vi "ABB Report Bearing run.vi"(10 "Report in":string) -> (2 "Report out":string)   [LabVIEW 2017]
uses:
  ABB global.vi
panel:
  out "Selected Entries":string[](array[string])
  out "appended array":string[][](array[string])
  out "subarray":dbl[](array[numeric])
  out "Bearing run":cluster{"Heat run results":dbl[], dbl[]}[](graph)
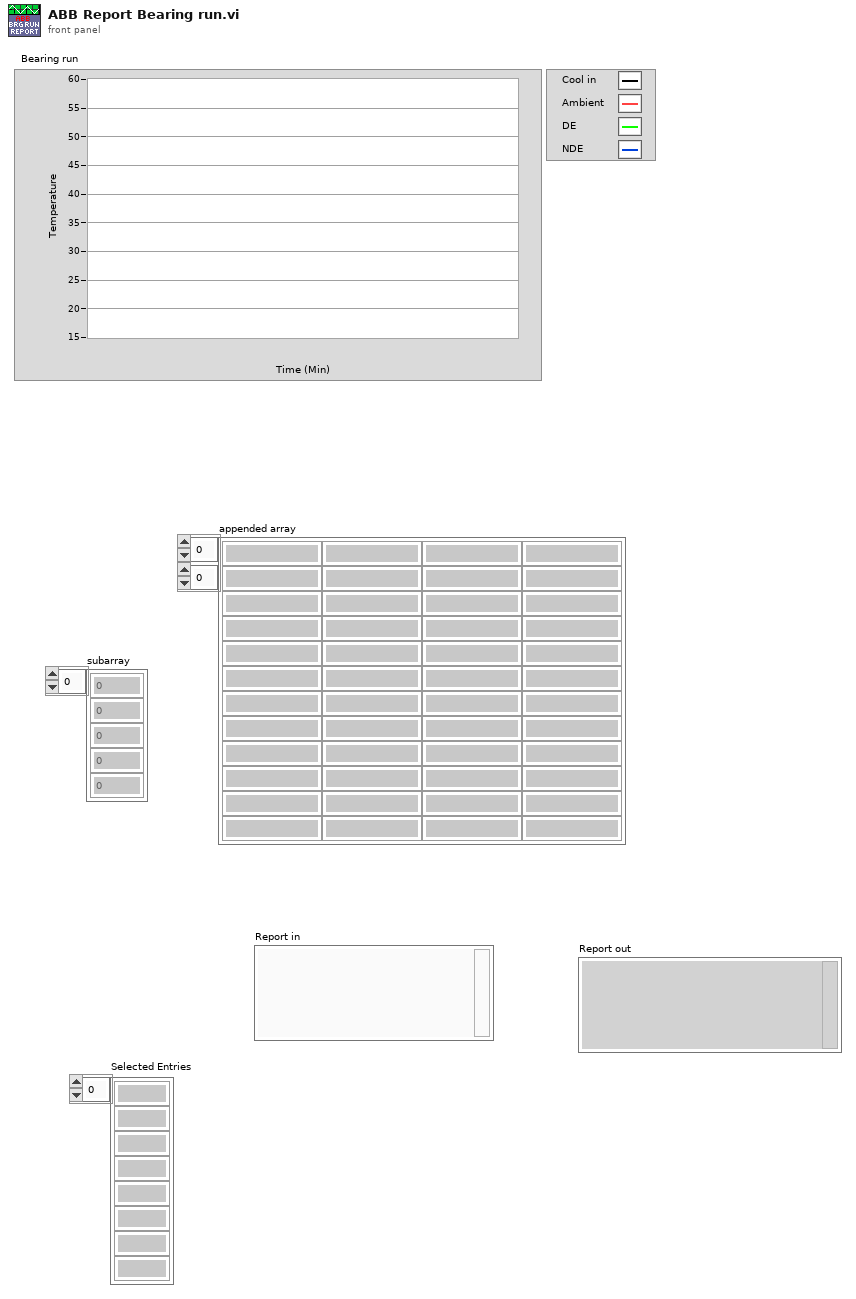
[diagram p1: front panel]
types:
  T1 = cluster{"temp. alloc":i32[], "category":i32[], "Category names":string[], "Category none names":string[]}
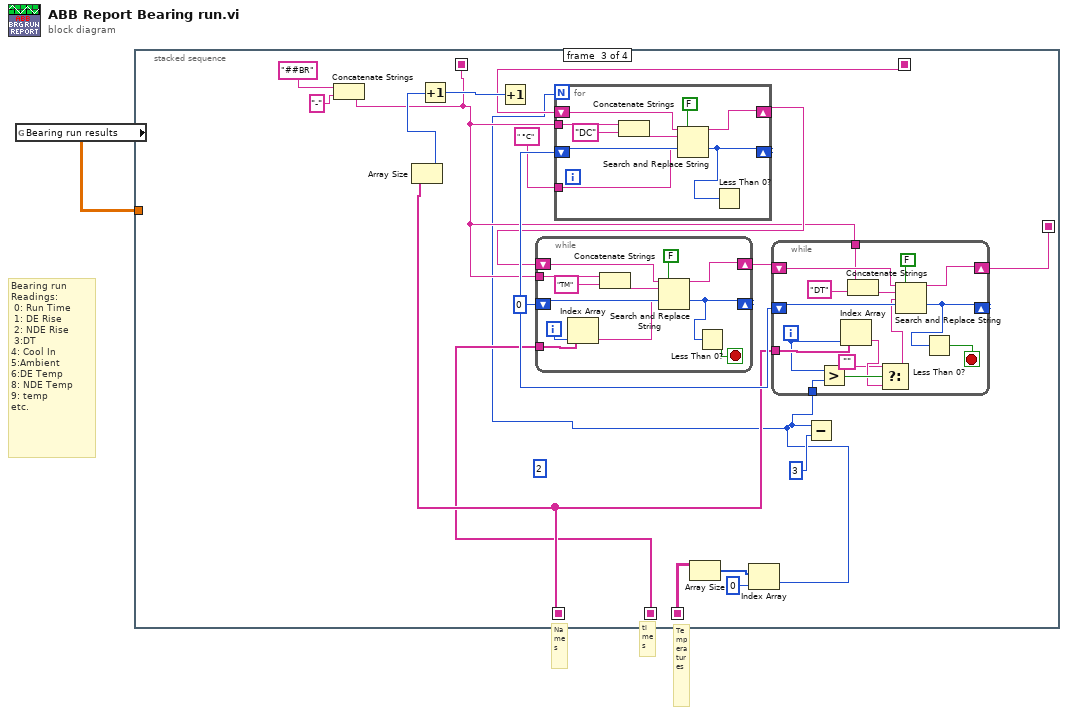
[diagram p0: block diagram]
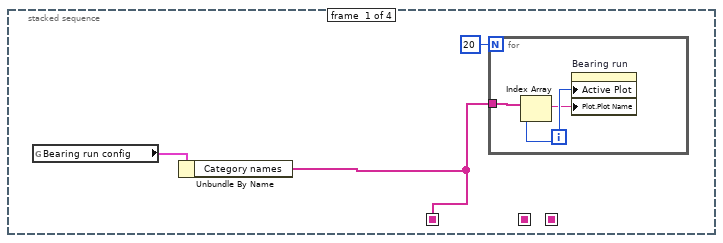
[diagram p2: hidden frame]
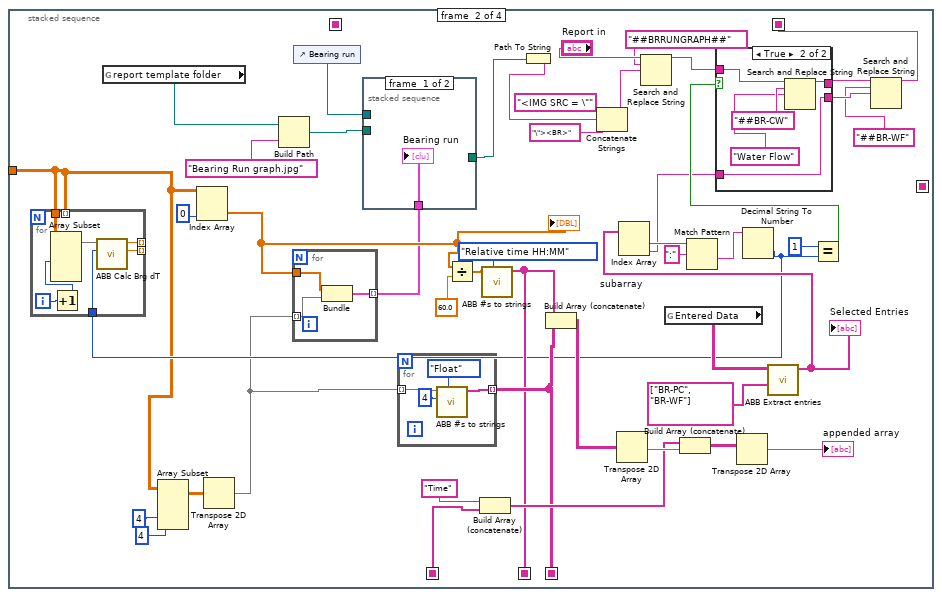
[diagram p3: hidden frame]
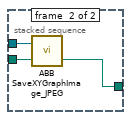
[diagram p4: hidden frame]
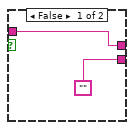
[diagram p5: hidden frame]
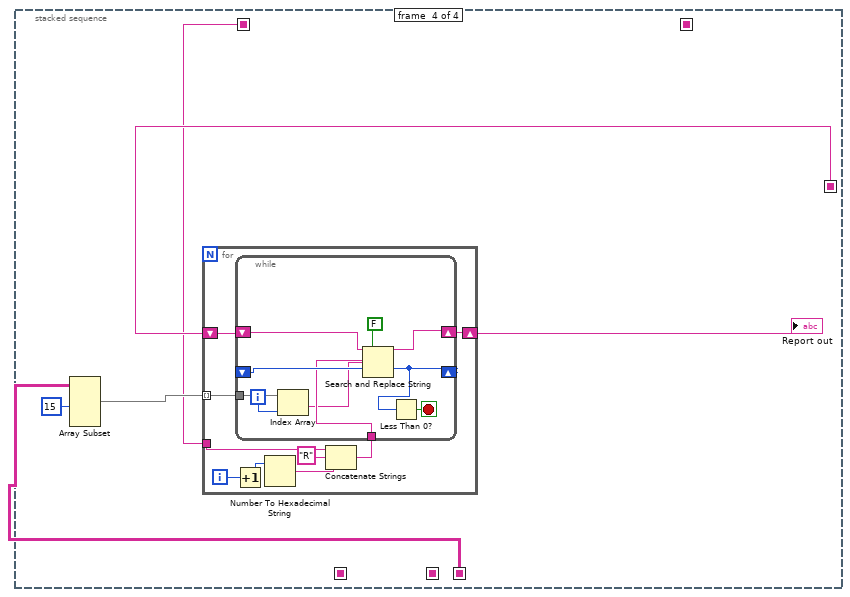
[diagram p6: hidden frame]
diagram:
  # "Bearing run Readings:\n 0: Run Time\n 1: DE Rise\n 2: NDE Rise\n 3:DT\n4: Cool In\n5:Ambient\n6:DE Temp\n8: NDE Temp\n9: temp\netc."
  # "Names"
  # "Temperatures"
  # "times"
  n1 = global read "ABB global.vi" "Bearing run results"() -> (w1:dbl[][])
  n2 = stacked-sequence {
    seq-local: [_ w22 _ _] -> [_ _ w87 _]
    seq-local: [_ w35 _ _] -> [_ _ w82 w135]
    seq-local: [w2 _ _ _] -> [_ w33 w86 _]
    seq-local: [_ w34 _ _] -> [_ _ w85 _]
    seq-local: [_ _ w83 _] -> [_ _ _ w136]
    seq-local: [_ _ w84 _] -> [_ _ _ w134]
    tunnel: w1 -> [_ w11 _ _]
    frame #0 {
      n3 = global read "ABB global.vi" "Bearing run config"() -> (w4:T1)
      n4 = Unbundle By Name(w4) -> ("Category names"=w2:string[])
      n5 = for {
        N: 20 -> [_]
        tunnel: w2 -> [w6]
        i -> [w7]
        n6 = Index Array(array=w6, index=w7) -> (element=w5:string)
        n7 = property on="Bearing run" class="XYGraph (strict)"("Active Plot"=w7, "Plot.Plot Name"=w5) -> ()  [unwired: 2 in, 2 out]
      }
    }
    frame #1 {
      n8 = global read "ABB global.vi" "report template folder"() -> (w44:path)
      n9 = Array Subset(array=w11, index (col)=4 ("index"), length (col)=4 ("length")) -> (w9:dbl[][])  [unwired: 2 in]
      n10 = Index Array(array=w11, index (col)=0 ("disabled index (col)")) -> (element=w16:dbl[])  [unwired: 1 in]
      "subarray" <- w16
      n11 = Transpose 2D Array(2D array=w9) -> (transposed array=w8:dbl[][])
      n12 = Build Path(base path=w44, name or relative path="Bearing Run graph.jpg") -> (appended path=w49:path)
      n13 = for {
        tunnel: w16 -> [w77]
        tunnel: w8 -> [w76] mode=indexing
        tunnel: [w75] -> w14 mode=indexing
        n14 = Bundle("Bearing run results"=w77, w76) -> (w75:cluster{"Bearing run results":dbl[], dbl[]})  [unwired: 1 in]
      }
      n15 = control-ref of="Bearing run"() -> (w53:refnum<vi>)
      n16 = stacked-sequence {
        tunnel: w53 -> [_ w63]
        tunnel: w49 -> [_ w62]
        tunnel: [_ w62] -> w15
        tunnel: w14 -> [w61 _]
        frame #0 {
          "Bearing run" <- w61
        }
        frame #1 {
          n17 = call "ABB SaveXYGraphImage_JPEG.vi"("Path"=w62, "COntrolReference"=w63) -> ()  [unwired: 2 in]
        }
      }
      n18 = for {
        tunnel: w8 -> [w74] mode=indexing
        tunnel: [w71] -> w35 mode=indexing
        n19 = call "ABB #s to strings.vi"("# type"=enum16{"Float", "Relative time HH:MM"}."Float", "Precision"=4, "Numbers in"=w74) -> ("Strings out"=w71:string[])  [unwired: 8 in]
      }
      n20 = Divide(x=w16, y=60.0) -> (x/y=w18:dbl[])
      n21 = Build Array (concatenate)("Time", w33) -> (w37:string[])
      n22 = call "ABB #s to strings.vi"("# type"=enum16{"Float", "Relative time HH:MM"}."Relative time HH:MM", "Numbers in"=w18) -> ("Strings out"=w34:string[])  [unwired: 9 in]
      n23 = Path To String(path=w15) -> (string=w48:string)
      n24 = Build Array (concatenate)(w34, w35) -> (w41:string[][])
      n25 = Concatenate Strings("<IMG SRC = \"", w48, "\"><BR>" ("string")) -> (w50:string)
      n26 = Transpose 2D Array(2D array=w41) -> (transposed array=w40:string[][])
      n27 = Search and Replace String(input string="Report in", search string="##BRRUNGRAPH##", replace string=w50) -> (result string=w25:string)  [unwired: 5 in, 3 out]
      n28 = global read "ABB global.vi" "Entered Data"() -> (w32:string[][])
      n29 = Build Array (concatenate)(w37, w40) -> (w39:string[][])
      n30 = Transpose 2D Array(2D array=w39) -> (transposed array=→"appended array":string[][])
      n31 = call "ABB Extract entries.vi"("Entry IDs"=string[] ["BR-PC", "BR-WF"], "Entry table in"=w32) -> ("Selected Entries"=w30:string[])  [unwired: 9 in]
      "Selected Entries" <- w30
      n32 = Index Array(array=w30) -> (element #1=w29:string, element #2=w20:string)  [unwired: 2 in]
      n33 = Match Pattern(string=w29, regular expression=":") -> (after substring=w27:string)  [unwired: 1 in, 3 out]
      n34 = Decimal String To Number(string=w27) -> (number=w13:i32)  [unwired: 2 in, 1 out]
      n35 = for {
        tunnel: w11 -> [_] mode=indexing
        tunnel: w11 -> [w57]
        tunnel: [w56] -> _ mode=indexing
        tunnel: [w55] -> _ mode=indexing
        tunnel: w13 -> [w54]
        i -> [w60]
        n36 = Increment(x=w60) -> (x+1=w59:i32)
        n37 = Array Subset(array=w57, length (row)=w59) -> (w58:dbl[][])  [unwired: 3 in]
        n38 = call "ABB Calc Brg dT.vi"("Primary coolant"=w54, "Readings in"=w58) -> ("NDE rise"=w55:dbl, "DE rise"=w56:dbl)  [unwired: 5 in, 3 out]
      }
      n39 = Equal?(x=1, y=w13) -> (x = y?=w24:bool)
      n40 = case shown="True" w24 {
        tunnel: w25 -> [w65 w70]
        tunnel: [w65 w67] -> w23
        tunnel: ["" w66] -> w21
        tunnel: w20 -> [_ w66]
        frame False {
        }
        frame True {
          n41 = Search and Replace String(input string=w70, search string="##BR-CW", replace string="Water Flow") -> (result string=w67:string)  [unwired: 5 in, 3 out]
        }
      }
      n42 = Search and Replace String(input string=w23, search string="##BR-WF", replace string=w21) -> (result string=w22:string)  [unwired: 5 in, 3 out]
    }
    frame #2 {
      (unwired) 2 ("y")
      w92 = 0 ("offset past replacement")
      n43 = Concatenate Strings("##BR" ("search string"), "-" ("string")) -> (w84:string)
      n44 = Array Size(array=w86) -> (size(s)=w89:i32)
      n45 = Increment(x=w89) -> (x+1=w88:i32)
      n46 = Increment(x=w88) -> ()  [unwired: 1 out]
      n47 = Array Size(array=w82) -> (size(s)=w81:i32[])
      n48 = Index Array(array=w81, index=0) -> (element=w78:i32)
      n49 = for {
        N: w78 -> [_]
        shift-right: [w119] -> w90
        shift-left: w87 -> [w120]
        shift-right: [w112] -> _
        shift-left: w92 -> [w118]
        tunnel: w84 -> [w116]
        tunnel: " °C" ("Unit") -> [w113]
        n50 = Concatenate Strings(w116, "DC" ("search string")) -> (w114:string)
        n51 = Search and Replace String(replace all?=FALSE ("replace all? (F)"), input string=w120, search string=w114, replace string=w113, offset=w118) -> (result string=w119:string, offset past replacement=w112:i32)  [unwired: 3 in, 2 out]
        n52 = Less Than 0?(x=w112) -> ()  [unwired: 1 out]
      }
      n53 = while {
        shift-right: [w131] -> w95
        shift-left: w90 -> [w132]
        tunnel: w85 -> [w126]
        shift-right: [w127] -> _
        shift-left: w92 -> [w130]
        tunnel: w84 -> [w124]
        i -> [w125]
        stop <- w128 stop-if-true
        n54 = Index Array(array=w126, index=w125) -> (element=w121:string)
        n55 = Concatenate Strings(w124, "TM" ("search string")) -> (w122:string)
        n56 = Search and Replace String(replace all?=FALSE ("replace all? (F)"), input string=w132, search string=w122, replace string=w121, offset=w130) -> (result string=w131:string, offset past replacement=w127:i32)  [unwired: 3 in, 2 out]
        n57 = Less Than 0?(x=w127) -> (x < 0?=w128:bool)
      }
      n58 = while {
        shift-right: [w110] -> w83
        shift-left: w95 -> [w111]
        tunnel: w86 -> [w106]
        shift-right: [w107] -> _
        shift-left: w92 -> [w109]
        tunnel: w84 -> [w105]
        tunnel: w78 -> [w100]
        i -> [w101]
        stop <- w102 stop-if-true
        n59 = Greater?(x=w101, y=w100) -> (0:w99:bool)
        n60 = Index Array(array=w106, index=w101) -> (element=w98:string)
        n61 = Concatenate Strings(w105, "DT" ("search string")) -> (w103:string)
        n62 = Select(t="", s=w99, f=w98) -> (s? t:f=w96:string)
        n63 = Search and Replace String(replace all?=FALSE ("replace all? (F)"), input string=w111, search string=w103, replace string=w96, offset=w109) -> (result string=w110:string, offset past replacement=w107:i32)  [unwired: 3 in, 2 out]
        n64 = Less Than 0?(x=w107) -> (x < 0?=w102:bool)
      }
      n65 = Subtract(x=w78, y=3) -> ()  [unwired: 1 out]
    }
    frame #3 {
      n66 = Array Subset(array=w135, length (row)=15 ("length")) -> (w138:string[][])  [unwired: 3 in]
      n67 = for {
        tunnel: w138 -> [w147] mode=indexing
        shift-right: [w145] -> w133
        shift-left: w136 -> [w146]
        tunnel: w134 -> [w140]
        i -> [w144]
        n68 = Increment(x=w144) -> (x+1=w143:i32)
        n69 = Number To Hexadecimal String(2:w143) -> (0:w141:string)  [unwired: 1 in]
        n70 = Concatenate Strings(w140, "R" ("search string"), w141) -> (w139:string)
        n71 = while {
          shift-right: [w156] -> w145
          shift-left: w146 -> [w157]
          shift-right: [w152] -> _
          shift-left: _ -> [w155]
          tunnel: w147 -> [w150]
          tunnel: w139 -> [w149]
          i -> [w151]
          stop <- w153 stop-if-true
          n72 = Index Array(array=w150, index=w151) -> (element=w148:string)
          n73 = Search and Replace String(replace all?=FALSE ("replace all? (F)"), input string=w157, search string=w149, replace string=w148, offset=w155) -> (result string=w156:string, offset past replacement=w152:i32)  [unwired: 3 in, 2 out]
          n74 = Less Than 0?(x=w152) -> (x < 0?=w153:bool)
        }
      }
      "Report out" <- w133
    }
  }
